vi "FS Operation Extrude.vi"(6 "Extrude #":i32=1, 8 "Ignore Inner Loops?":bool=TRUE, 9 "Extrude Depth":dbl=1.5, 10 "Sketch # to Extrude":i32=1, 11 "Feature In":string="FeatureScript 1247;\nimport(path : \"onshape/std/geometry.fs\", version : \"1247.0\");\n\nannotation { \"Feature Type Name\" : \"LabVIEW Feature\" }\nexport const myFeature = defineFeature(function(context is Context, id is Id, definition is map)\n    precondition\n    {\n        // Define the parameters of the feature type\n    }\n    {\n        // Define the function's action\n    });") -> (3 "Feature Out":string="FeatureScript 1247;\nimport(path : \"onshape/std/geometry.fs\", version : \"1247.0\");\n\nannotation { \"Feature Type Name\" : \"LVFeat1\" }\nexport const myFeature = defineFeature(function(context is Context, id is Id, definition is map)\n    precondition\n    {\n        // Define the parameters of the feature type\n    }\n    {\n        // Define the function's action\n\nvar sketch1 = newSketch(context, id + \"sketch1\", {\n                \"sketchPlane\" : qCreatedBy(makeId(\"Top\"), EntityType.FACE)\n        });\n        // Create sketch entities here\n        skRectangle(sketch1, \"rectangle1\", {\n                \"firstCorner\" : vector(0, 0) * inch,\n                \"secondCorner\" : vector(3, 4) * inch\n        });\n        \n        skSolve(sketch1);\n    });")   [LabVIEW 2019]
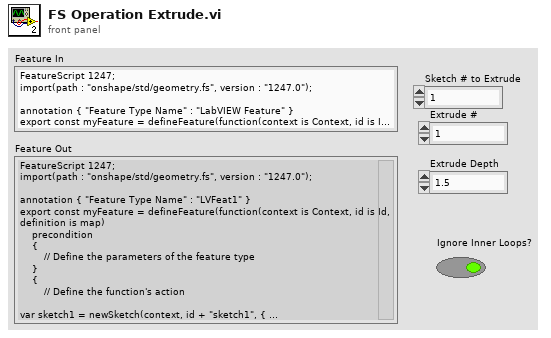
[diagram p1: front panel]
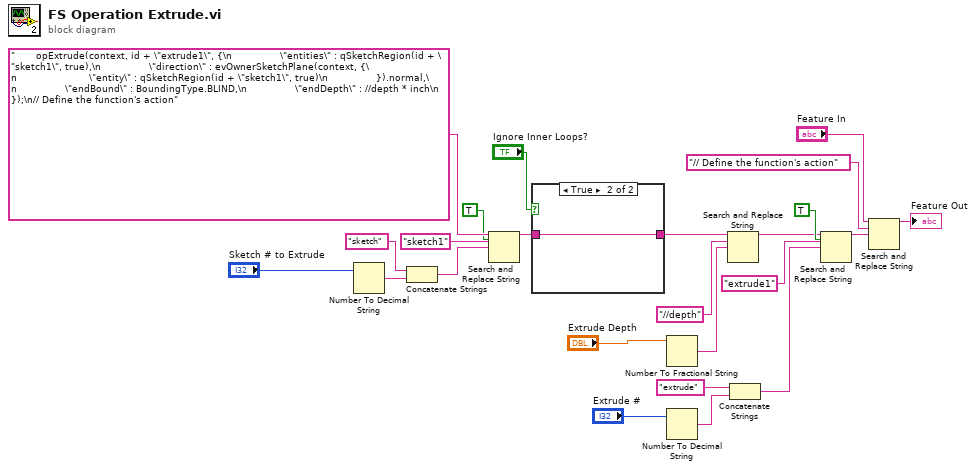
[diagram p0: block diagram]
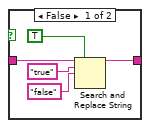
[diagram p2: hidden frame]
diagram:
  n1 = Number To Decimal String(number="Sketch # to Extrude") -> (decimal integer string=w13:string)  [unwired: 1 in]
  n2 = Concatenate Strings("sketch" ("regular expression"), w13) -> (w10:string)
  n3 = Search and Replace String(replace all?=TRUE ("replace all? (F)"), input string="       opExtrude(context, id + \"extrude1\", {\n                \"entities\" : qSketchRegion(id + \"sketch1\", true),\n                \"direction\" : evOwnerSketchPlane(context, {\n                        \"entity\" : qSketchRegion(id + \"sketch1\", true)\n                }).normal,\n                \"endBound\" : BoundingType.BLIND,\n                \"endDepth\" : //depth * inch\n        });\n// Define the function's action" ("search string"), search string="sketch1" ("regular expression"), replace string=w10) -> (result string=w6:string)  [unwired: 4 in, 3 out]
  n4 = case shown="True" "Ignore Inner Loops?" {
    tunnel: [w25 w30] -> w4
    tunnel: w6 -> [w26 w30]
    frame False {
      n5 = Search and Replace String(replace all?=TRUE ("replace all? (F)"), input string=w26, search string="true" ("regular expression"), replace string="false" ("replace string (\"\")")) -> (result string=w25:string)  [unwired: 4 in, 3 out]
    }
    frame True {
    }
  }
  n6 = Number To Fractional String(number="Extrude Depth") -> (F-format string=w2:string)  [unwired: 3 in]
  n7 = Number To Decimal String(number="Extrude #") -> (decimal integer string=w14:string)  [unwired: 1 in]
  n8 = Search and Replace String(input string=w4, search string="//depth", replace string=w2) -> (result string=w3:string)  [unwired: 5 in, 3 out]
  n9 = Concatenate Strings("extrude" ("regular expression"), w14) -> (w18:string)
  n10 = Search and Replace String(replace all?=TRUE ("replace all? (F)"), input string=w3, search string="extrude1" ("regular expression"), replace string=w18) -> (result string=w8:string)  [unwired: 4 in, 3 out]
  n11 = Search and Replace String(input string="Feature In", search string="// Define the function's action", replace string=w8) -> (result string=→"Feature Out":string)  [unwired: 5 in, 3 out]
